vi "ICPCON Read.vi"(8 "error in (no error)":errorcluster caption="错误输入（无错误）", 9 "Last Data Array":dbl[](array[numeric])=[0.0, 0.0, 0.0, 0.0, 0.0, 0.0, 0.0, 0.0] caption="原数据数组", 10 "write buffer":string caption="写入缓冲区", 11 "VISA Ref Input":refnum<visa-resource-name>="COM1" caption="VISA引用句柄输入") -> (0 "error out":errorcluster caption="错误输出", 1 "New Data Array":dbl[](array[numeric]) caption="新数据数组", 3 "VISA Ref Output":refnum<visa-resource-name> caption="VISA引用句柄输出")   [LabVIEW 2015]
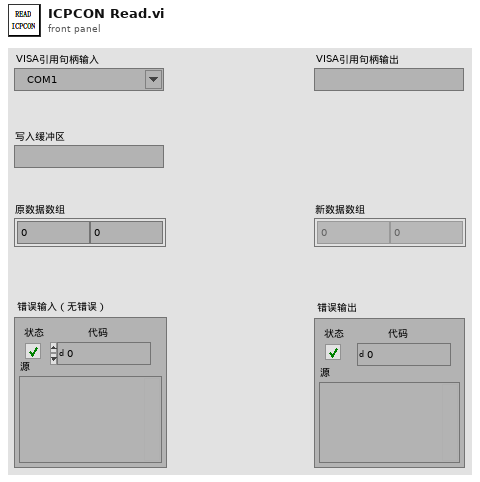
[diagram p1: front panel]
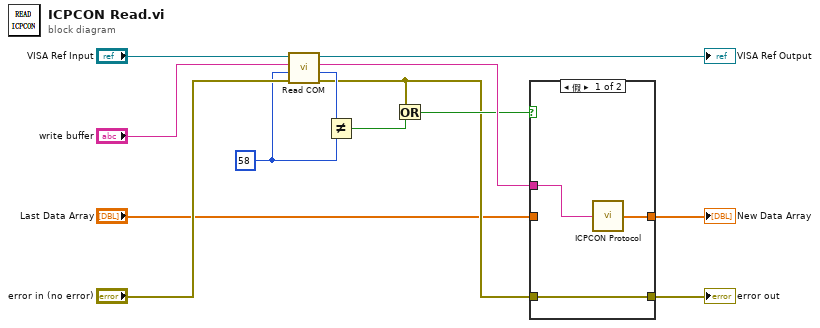
[diagram p0: block diagram]
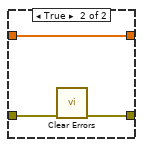
[diagram p2: hidden frame]
diagram:
  w6 = u32 58 ("read bytes")
  n1 = call "Read COM.vi"("error in"="error in (no error)", "read bytes"=w6, "write to buffer"="write buffer", "VISA resource name in"="VISA Ref Input") -> ("error out"=w2:errorcluster, "get bytes"=w7:u32, "read from buffer"=w10:string, "VISA resource name out"=→"VISA Ref Output":refnum<visa-resource-name>)  [unwired: 4 in]
  n2 = Not Equal?(x=w7, y=w6) -> (x != y?=w5:bool)
  n3 = Or(x=w2, y=w5) -> (x .or. y?=w4:bool)
  n4 = case shown="假" w4 {
    tunnel: [w16 w17] -> w13
    tunnel: w10 -> [w15 _]
    tunnel: w2 -> [w14 w19]
    tunnel: [w14 w18] -> w3
    tunnel: "Last Data Array" -> [_ w17]
    frame False {
      n5 = call "ICPCON Protocol.vi"("read buffer"=w15) -> ("Data Array"=w16:dbl[])
    }
    frame True {
      n6 = call <vilib>:"Clear Errors.vi"("error in (no error)"=w19) -> ("error out"=w18:errorcluster)  [unwired: 5 in, 1 out]
    }
  }
  "New Data Array" <- w13
  "error out" <- w3
